vi "Init Attributes.vi"(10 "Attributes":T1) -> (2 "Attributes":refnum<class "Attributes.lvclass">)   [LabVIEW 2020, in "jettl.lvlib" / "Base Attributes.lvlib"]
uses:
  Base Attributes.lvlib
  Attributes/Attributes.lvclass
  Attributes.ctl
  Transport/Transport.lvclass
  Msgs.ctl
  Msg/Msg.lvclass
  Actor/Actor.lvclass
  Base Attributes/Base Attributes.lvclass/Base Attributes.ctl
  Base Attributes/Base Attributes.lvclass
  C:/git/jettl/src/jettl/jettl/Attributes/Attributes.lvclass
  jettl.lvlib
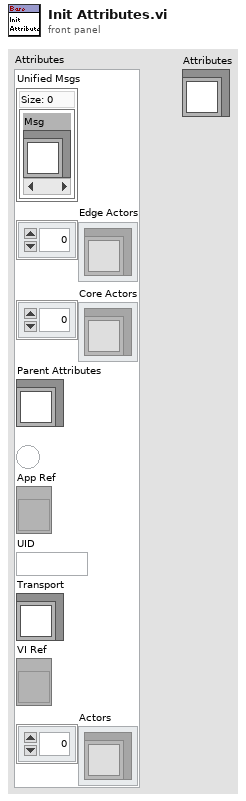
[diagram p1: front panel]
types:
  T1 = typedef "jettl.lvlib/Attributes.ctl" = cluster{"Unified Msgs":T2, "Edge Actors":refnum<class "Actor.lvclass">[], "Core Actors":refnum<class "Actor.lvclass">[], "Parent Attributes":refnum<class "Attributes.lvclass">, "Root":bool, "App Ref":refnum<vi>, "UID":string, "Transport":refnum<class "Transport.lvclass">, "VI Ref":refnum<vi>, "Actors":refnum<class "Actor.lvclass">[]}
  T2 = typedef "jettl.lvlib/Msgs.ctl" = set{refnum<class "Msg.lvclass">}
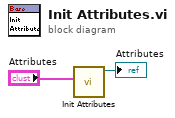
[diagram p0: block diagram]
diagram:
  n1 = call "Init Attributes.vi"("Attributes"="Attributes") -> ("Base Attributes out"=→"Attributes":refnum<class "Base Attributes.lvclass">)  [unwired: 10 in]
